vi "EOL CAN_Get Vehicle type.vi"(7 "Rx Arbitration Id":u32=402522244 format="%.0x", 8 "error in (no error)":errorcluster, 9 "Tx Arbitration Id":u32=402391172 format="%.0x", 10 "Read Session in":refnum<k21>, 11 "Write Session in":refnum<k21>) -> (0 "error out":errorcluster, 2 "Vehicle Type":string, 3 "Response Good?":bool, 5 "TxRx Data":string[][](array[string]))   [LabVIEW 2018]
uses:
  <vilib>/xnet/xnet.llb/XNET Frame CAN.ctl
  <vilib>/xnet/xnet.llb/XNET Frame Type CAN.ctl
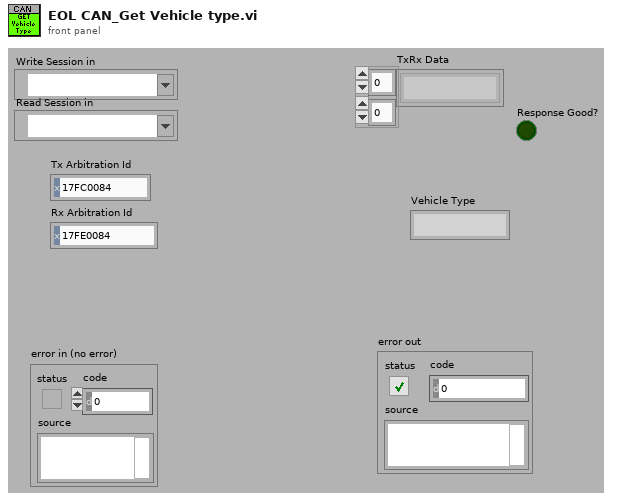
[diagram p1: front panel]
types:
  T1 = typedef "XNET Frame CAN.ctl" = cluster{"timestamp":timestamp, "payload":u8[], "identifier":u32, "type":T2, "extended?":bool, "echo?":bool}
  T2 = typedef "XNET Frame Type CAN.ctl" = u8
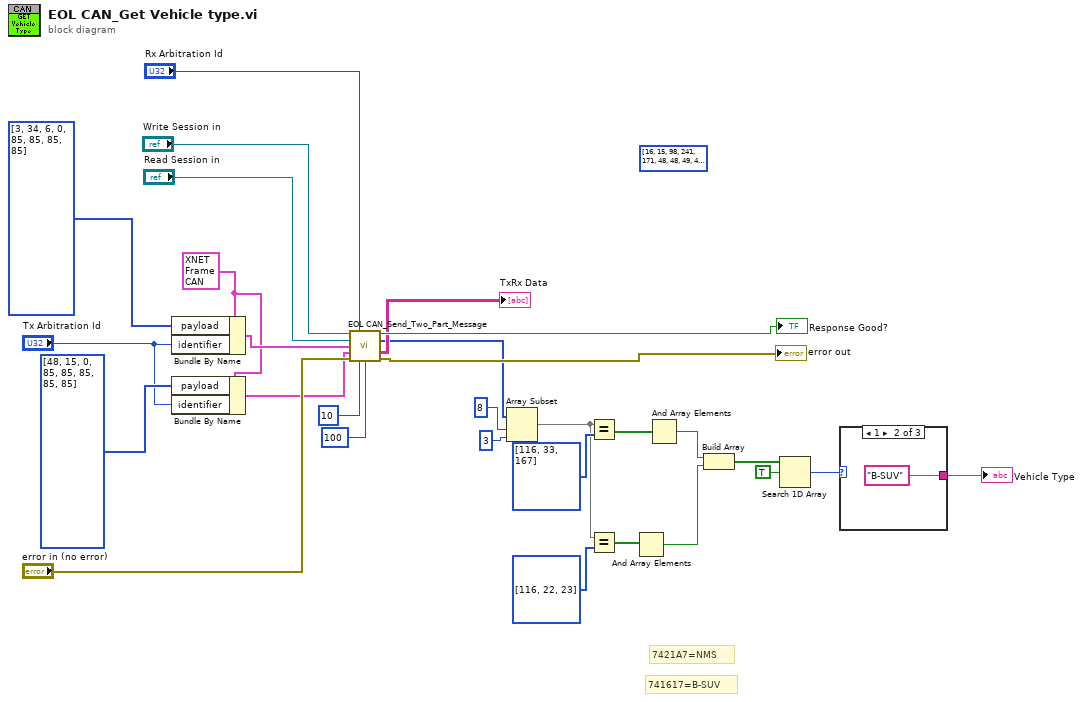
[diagram p0: block diagram]
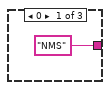
[diagram p2: hidden frame]
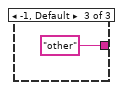
[diagram p3: hidden frame]
diagram:
  w17 = T1 {"timestamp"=timestamp(0 s since 1904-01-01), "payload"=[2, 39, 3, 85, 85, 85, 85, 85], "identifier"=402391172, "type"=0, "extended?"=TRUE, "echo?"=FALSE} ("Tx CAN frame 1")
  (unwired) u8[] [16, 15, 98, 241, 171, 48, 48, 49, 48, 48, 48, 48, 53, 48, 48, 48, 51, 170, 170, 170, 170, 170] ("Rx Data")
  # "741617=B-SUV"
  # "7421A7=NMS"
  n1 = Bundle By Name(cluster=w17, "payload"=u8[] [3, 34, 6, 0, 85, 85, 85, 85] ("Transmit Data"), "identifier"="Tx Arbitration Id") -> (w18:T1)
  n2 = Bundle By Name(cluster=w17, "payload"=u8[] [48, 15, 0, 85, 85, 85, 85, 85] ("Transmit Data"), "identifier"="Tx Arbitration Id") -> (w16:T1)
  n3 = call "EOL CAN_Send_Two_Part_Message.vi"("Write Session in"="Write Session in", "Rx Arbitration Id"="Rx Arbitration Id", "Read Session in"="Read Session in", "Tx CAN frame 1"=w18, "Tx CAN frame 2"=w16, "error in (no error)"="error in (no error)", "Retries"=10, "Msg Wait Time"=u32 100) -> ("Response Good?"=→"Response Good?":bool, "Rx Data"=w23:u8[], "TxRx Data"=→"TxRx Data":string[][], "error out"=→"error out":errorcluster)  [unwired: 4 in]
  n4 = Array Subset(array=w23, index=8, length=3) -> (w8:u8[])
  n5 = Equal?(x=w8, y=u8[] [116, 33, 167]) -> (x = y?=w10:bool[])
  n6 = Equal?(x=w8, y=u8[] [116, 22, 23]) -> (x = y?=w7:bool[])
  n7 = And Array Elements(Boolean array=w7) -> (logical AND=w5:bool)
  n8 = And Array Elements(Boolean array=w10) -> (logical AND=w6:bool)
  n9 = Build Array(w6, w5) -> (w4:bool[])
  n10 = Search 1D Array(1D array=w4, element=TRUE) -> (index of element=w2:i32)  [unwired: 1 in]
  n11 = case shown="1" w2 {
    tunnel: ["NMS" ("type") "B-SUV" ("type") "other" ("type")] -> w1
    frame 0 {
    }
    frame 1 {
    }
    frame -1, Default {
    }
  }
  "Vehicle Type" <- w1
